vi "PH_Sequencer.SCR Enable Sub-GDs.vi"(0 "i ref in":refnum<vi>, 5 "error in (no error)":errorcluster) -> (14 "i ref out":refnum<vi>, 19 "error out":errorcluster)   [LabVIEW 2014, in "PH_Sequencer.lvlib"]
doc: "This VI sends a state change request to the Seq SM. If the sequencer is in state \"Start Fast Devices\", and all PPMA PUs which are in use are in state PU SM \"Switch GD Channel on\", \"Enable Sub-GDs\" is requested."
uses:
  PH_Sequencer.lvlib
  PH_PowerUnit_BaseClass/PH_PowerUnit_BaseClass.SM States.ctl
  CSCore/BaseSM/BaseSM.lvlib
  PH_BeamlineInformation/PH_BeamlineInformation.lvlib
  PH_PowerUnit_BaseClass/PH_PowerUnit_BaseClass.lvlib
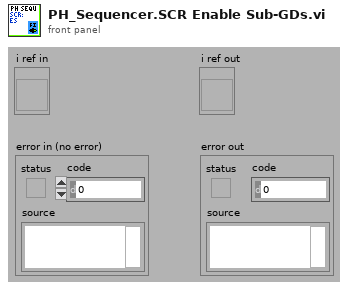
[diagram p1: front panel]
types:
  T1 = typedef "PH_PowerUnit_BaseClass.lvlib/PH_PowerUnit_BaseClass.SM States.ctl" = enum16{".", "Stand by", "Switch PU on", "Configure", "Set Default Voltage", "Set STANDBY", "Set READY", "Wait for Shot Cmd", "Open Dump Rods", "Open Ross Relais", "Close Ross Relais", "Switch PSU on", "Switch PSU off", "Charge", "Switch GD Channel on", "Close Dump Rods", "Rods-TO", "RR-TO", "PSU-TO", "Trigger-TO"}
  T2 = typedef "PH_BeamlineInformation.lvlib/PH_BeamlineInformation.i attribute.ctl" = cluster{"BL GUI Elements of Services":cluster{"Service Name":string, "GUI Elements":refnum<vi>[], "Status":i32}[], "Powermeters":T3, "Efficiency":T4, "Heads":T5[]}
  T3 = typedef "PH_BeamlineInformation.lvlib/PH_BeamlineInformation.Powermeter.ctl" = cluster{"ns FE":cluster{"GUI Ref":refnum<vi>, "Value":dbl}, "fs FE":cluster{"GUI Ref":refnum<vi>, "Value":dbl}, "PA":cluster{"GUI Ref":refnum<vi>, "Value":dbl}, "MA":cluster{"GUI Ref":refnum<vi>, "Value":dbl}, "Z6 green":cluster{"GUI Ref":refnum<vi>, "Value":dbl}, "Z6 IR":cluster{"GUI Ref":refnum<vi>, "Value":dbl}, "Z6 COS":cluster{"GUI Ref":refnum<vi>, "Value":dbl}}
  T4 = typedef "PH_BeamlineInformation.lvlib/PH_BeamlineInformation.Efficiency.ctl" = cluster{"PA Gain":cluster{"GUI Ref":refnum<vi>, "Value":dbl}, "MA Gain":cluster{"GUI Ref":refnum<vi>, "Value":dbl}, "Z6 green Conversion":cluster{"GUI Ref":refnum<vi>, "Value":dbl}, "Z6 Comp Losses":cluster{"GUI Ref":refnum<vi>, "Value":dbl}}
  T5 = typedef "PH_BeamlineInformation.lvlib/PH_BeamlineInformation.Head.ctl" = cluster{"PowerUnit":T6, "in use":cluster{"Value":bool, "GUI Ref":refnum<vi>, "linked":bool}, "voltage":cluster{"Value":dbl, "GUI Ref":refnum<vi>, "linked":bool}}
  T6 = typedef "PH_PP_Common.lvlib/PH_PP_Common.PUs.ctl" = enum16{"no Info", "PA-19mm-1", "PA-19mm-2", "PA-45mm-PILC", "PA-45mm-MAIN", "MA-PU-1", "MA-PU-2", "MA-PU-3", "MA-PU-4", "MA-PU-5", "MA-PU-6", "MA-FR", "MA-PILC", "PA-45mm-DP"}
  T7 = typedef "PH_Sequencer.lvlib/PH_Sequencer.i attribute.ctl" = cluster{"GUI Refs":cluster{"Main Off":refnum<vi>, "Fire":refnum<vi>, "Status":refnum<vi>, "Ready":refnum<vi>, "Waiting Time":refnum<vi>, "Timeout":refnum<vi>, "PPMA Ready":refnum<vi>, "Sequencer SM State":refnum<vi>, "PPPA Ready":refnum<vi>, "Calorimeter":refnum<vi>, "Beamline Ready":refnum<vi>, "Clear Beamline":refnum<vi>, "Linkage PPMA Rods":refnum<vi>, "Linkage Current PA":refnum<vi>, "Linkage Current MA":refnum<vi>, "Timing Ready":refnum<vi>, "State Timing":refnum<vi>, "Force Timing":refnum<vi>, "PSDB Shot Comment":refnum<vi>, "State PA Backreflection":refnum<vi>, "Beamline Z6 Ready":refnum<vi>, "Clear Z6 Beamline":refnum<vi>, "Sequence length":refnum<vi>, "Timing Mode":refnum<vi>, "Slow Trigger Settings":refnum<vi>, "Experiment Description":refnum<vi>, "State PSDB":refnum<vi>, "PSDB Ready":refnum<vi>, "Set PSDB Settings":refnum<vi>, "Get PSDB Info":refnum<vi>, "Take Snapshot":refnum<vi>, "Shottype":refnum<vi>, "Experiment":refnum<vi>, "Phase Frontends":refnum<vi>, "PP 45mm PILC in use":refnum<vi>}, "Status Info":cluster{"Machine Status":T8, "WaitingTime":i32, "Timeout":bool}, "Readyness":cluster{"Ready to shot":bool, "PPMA Ready":bool, "PPPA Ready":bool, "BL Ready":bool, "Timing Ready":bool, "BL Z6 Ready":bool, "PSDBReady":bool}, "Instancenames":cluster{"PPMA Rods":string, "PP Current Meas":string, "PH Beamline Chief":string, "PA Backrefl Meas":string, "Z6 Beamline Chief":string}, "Data to read":bool, "Calorimeter":cluster{"Instancename":string, "On":bool, "linked":bool}, "Linkage":cluster{"PPMA Rods":bool, "PP Current Meas":bool, "PHELIX Beamline Chief":bool, "PA Backrefl Meas":bool, "Z6 Beamline Chief":bool}, "Timing":cluster{"Instance":string, "linked":bool, "Status":T8, "Timing Mode":T9, "Slow Trigger Settings":T10, "Info available":cluster{"ext SlowTrigger":bool, "T2":bool, "Mode":bool, "Delay Slow Trigger":bool, "Phase FEs":bool}, "FE Phase":T11}, "Service ID R2S":i32, "PSDB":cluster{"Controller Instance":string, "Controller Status":T8, "Controller linked":bool, "Settings acknowledged":bool, "Current Experiment ID":i16, "Current Shot Type":i16, "Current Comment":string, "Remember Settings":bool, "Write 2 early":bool}, "PSDB Data":cluster{"Main Off?":bool, "Sequence Length":dbl, "Sequence startet":timestamp}, "6P 4Q Positions":cluster{"Instancename":string, "linked":bool, "Position":T12}[], "PUs":T13[]}
  T8 = typedef "PH_StatusHandler.lvlib/PH_StatusHandler.Status.ctl" = i16
  T9 = typedef "PH_Timing.lvlib/PH_Timing.Timing Mode.ctl" = cluster{"T2":i16, "Modeselector":enum32{"10 Hz", "0.5 Hz", "Shot"}}
  T10 = typedef "PH_Timing.lvlib/PH_Timing.Slow Trigger Settings.ctl" = cluster{"Delay":dbl, "externally triggered?":bool}
  T11 = typedef "PH_Timing.lvlib/PH_Timing.Phase FEs.ctl" = cluster{"Phase":dbl}
  T12 = typedef "PH_4_Pos_Selector.lvlib/PH_4_Pos_Selector.Position Selector.ctl" = u16
  T13 = typedef "PH_Sequencer.lvlib/PH_Sequencer.Head.ctl" = cluster{"PowerUnit":T6, "GUI Ref":refnum<vi>, "Information":T14, "linked?":bool, "GUI Ref Current Voltage":refnum<vi>}
  T14 = typedef "PH_Sequencer.lvlib/PH_Sequencer.PU Information.ctl" = cluster{"State":T8, "Waiting Time [s]":dbl, "PU State SM":T1, "PU Timeout SM":T1}
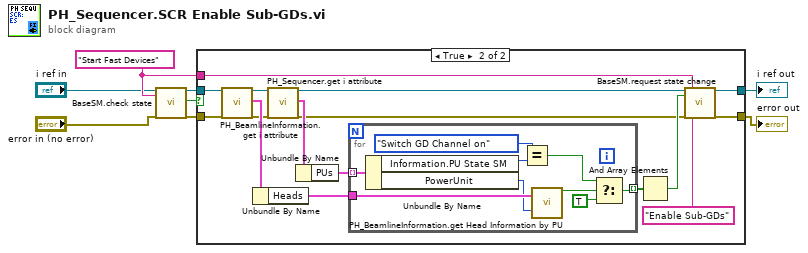
[diagram p0: block diagram]
diagram:
  w8 = "Start Fast Devices" ("requested state")
  n1 = call "BaseSM.check state.vi"("i ref in"="i ref in", "requestedState"=w8, "error in (no error)"="error in (no error)") -> ("i ref out"=w2:refnum<vi>, "OK"=w1:bool, "error out"=w3:errorcluster)  [unwired: 11 in, 3 out]
  n2 = case shown="True" w1 {
    tunnel: w8 -> [_ w26]
    tunnel: [w9 w24] -> w7
    tunnel: [w10 w23] -> w6
    tunnel: w3 -> [w9 w20]
    tunnel: w2 -> [w10 w21]
    frame False {
    }
    frame True {
      n3 = call "PH_BeamlineInformation.get i attribute.vi"("i ref in"=w21, "error in (no error)"=w20) -> ("i ref out"=w16:refnum<vi>, "i attribute"=w18:T2, "error out"=w14:errorcluster)  [unwired: 15 in]
      n4 = Unbundle By Name(w18) -> ("Heads"=w12:T5[])
      n5 = call "PH_Sequencer.get i attribute.vi"("i ref in"=w16, "error in (no error)"=w14) -> ("i ref out"=w15:refnum<vi>, "i attribute"=w17:T7, "error out"=w13:errorcluster)  [unwired: 15 in]
      n6 = Unbundle By Name(w17) -> ("PUs"=w11:T13[])
      n7 = for {
        tunnel: [w29] -> w19 mode=indexing
        tunnel: w12 -> [w35]
        tunnel: w11 -> [w34] mode=indexing
        n8 = Unbundle By Name(w34) -> ("Information.PU State SM"=w31:T1, "PowerUnit"=w33:T6)
        n9 = Equal?(x=PH_PowerUnit_BaseClass.SM_States."Switch GD Channel on", y=w31) -> (x = y?=w28:bool)
        n10 = call "PH_BeamlineInformation.get Head Information by PU.vi"("Heads"=w35, "Power Unit"=w33) -> ("In Use?"=w32:bool)  [unwired: 12 in, 5 out]
        n11 = Select(t=w28, s=w32, f=TRUE) -> (s? t:f=w29:bool)
      }
      n12 = And Array Elements(Boolean array=w19) -> (logical AND=w22:bool)
      n13 = call "BaseSM.request state change.vi"("i ref in"=w15, "change"=w22, "error in (no error)"=w13, "allowed current state"=w26, "requested state"="Enable Sub-GDs" ("next state")) -> ("i ref out"=w23:refnum<vi>, "error out"=w24:errorcluster)  [unwired: 11 in, 2 out]
    }
  }
  "error out" <- w7
  "i ref out" <- w6
